vi "Handle Connection.vi"(8 "error in (no error)":errorcluster, 10 "Client URI":refnum<class "URI.lvclass">, 11 "Connection Handler in":refnum<class "Connection Handler.lvclass">) -> (0 "error out":errorcluster, 2 "Close?":bool)   [LabVIEW 2020, in "HTTP Server.lvlib" / "Connection Handler.lvclass"]
uses:
  Connection Handler.lvclass
  lv-uri/URI/URI/URI.lvclass
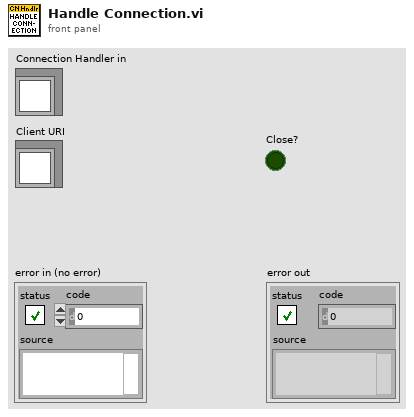
[diagram p1: front panel]
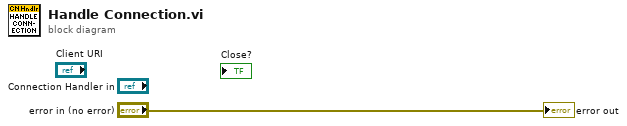
[diagram p0: block diagram]
diagram:
  "error out" <- "error in (no error)"
